vi "CRYPEAQ Global.vi"() -> ()   [LabVIEW 2013]
panel:
  out "Fmem.Adap.Rd":dbl[](array[numeric]) format="%.2f"
  out "Fmem.Adap.PC":dbl[][](array[numeric]) format="%.2f"
  out "Fmem.Adap.P":dbl[][](array[numeric]) format="%.2f"
  out "Fmem.Adap.Rn":dbl[](array[numeric]) format="%.2f"
  out "Fmem.TDS.Ef":dbl[][](array[numeric]) format="%.2f"
  out "Fmem.Env.Ese":dbl[][](array[numeric]) format="%.2f"
  out "Fmem.Env.DE":dbl[][](array[numeric]) format="%.2f"
  out "Fmem.Env.Eavg":dbl[][](array[numeric]) format="%.2f"
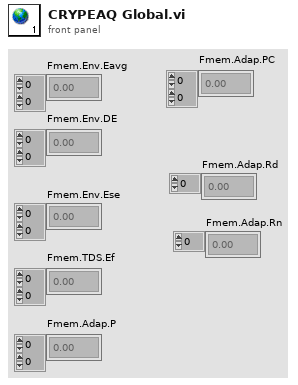
[diagram p1: front panel]
diagram:
